vi "Autonomous Independent.vi"() -> ()   [LabVIEW 2023]
doc: "This VI is called when autonomous begins, and will automatically be terminated when autonomous ends. You can carry out timed or sensor driven robot movement independently without needing to return to the caller."
uses:
  <vilib>/Rock Robotics/WPI/ThirdParty/REV Robotics/REVLib/Typedef/Spark MAX Idle Mode.ctl
  <vilib>/Rock Robotics/WPI/SafetyOutput/WPI_SafetyOutputConfigMenu.ctl
  <vilib>/Rock Robotics/Network Tables/NT Read String.vi
  <vilib>/Rock Robotics/WPI/Utilities/WPI_GetSetVariantRefNum.vi
panel:
  out "Numeric 2":i32
  in  "Numeric":i32
  out "Sensor Position 8":dbl
  out "Sensor Position 7":dbl
  out "?":dbl
  out "Sensor Position 6":dbl
  out "Sensor Position 5":dbl
  out "Sensor Position 4":dbl
  out "Sensor Position 3":dbl
  out "Sensor Position 2":dbl
  out "Sensor Position":dbl
  out "?":dbl
  # "Autonomous Independent.viBe sure to right-click and choose Data Operations>>Make Current Value default if you want to save the array values with the VI"
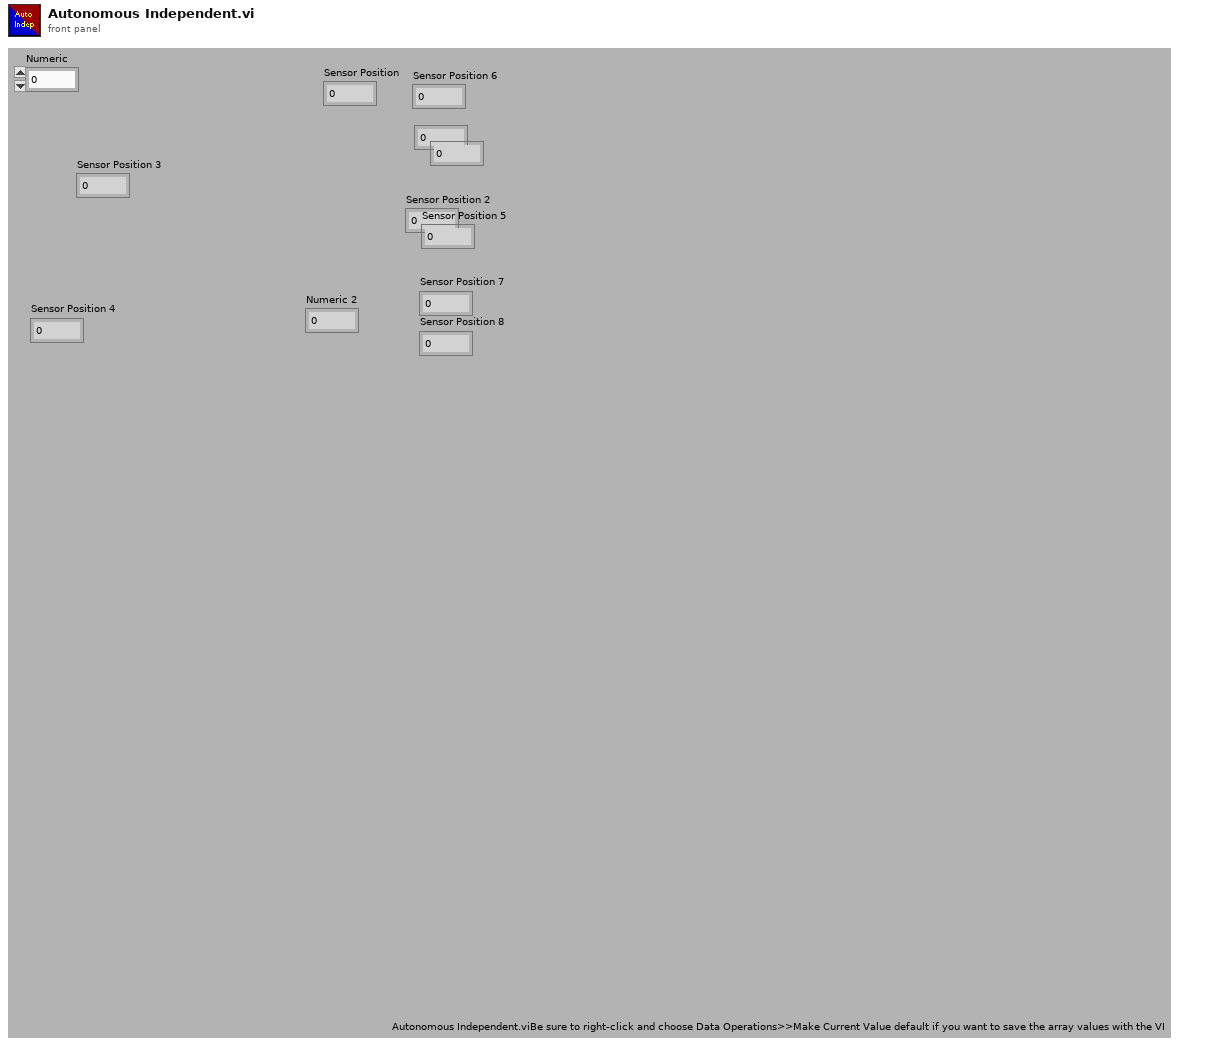
[diagram p1: front panel]
types:
  T1 = typedef "WPI_SafetyOutputConfigMenu.ctl" = enum16{"Enable", "Disable"}
  T2 = enum16{"ação 1", "ação 2", "ação 3", "ação 4", "ação 5", "ação 7", "ação 8"}
  T3 = typedef "Spark MAX Idle Mode.ctl" = enum16{"Coast", "Brake"}
  T4 = enum16{"ação 1", "ação 2", "ação 3", "ação 4", "ação 5"}
  T5 = typedef "WPI_RobotDriveDevRef.ctl" = cluster{"DevStatus":errorcluster, "Motors[]":T6[], "Square Inputs":bool, "Max Output":dbl}
  T6 = typedef "WPI_MotorControlDeviceRef.ctl" = cluster{"DeviceStatus":errorcluster, "Type":T7, "PWM":cluster{"PWM Channel":T8, "DeadBand":T9}, "CAN":cluster{"Device Number":u8, "SetOutput VI Ref":variant, "GetOutput VI Ref":variant, "Enable VI Ref":variant, "Disable VI Ref":variant, "Data":variant}, "Invert":bool, "DIO PWM":cluster{"PWM \"Enable\" Channel":T8, "DIOChannel":T10, "PWM Rate":dbl}}
  T7 = typedef "WPI_MotorControlType.ctl" = enum16{"PWM", "CAN", "DIO PWM"}
  T8 = typedef "FPGA_DIOPWMChannel.ctl" = enum8{"PWM 0", "PWM 1", "PWM 2", "PWM 3", "PWM 4", "PWM 5", "PWM 6", "PWM 7", "PWM 8", "PWM 9", "PWM MXP 0", "PWM MXP 1", "PWM MXP 2", "PWM MXP 3", "PWM MXP 4", "PWM MXP 5", "PWM MXP 6", "PWM MXP 7", "PWM MXP 8", "PWM MXP 9", "Invalid"}
  T9 = typedef "WPI_PWMDeadband.ctl" = cluster{"Name":string, "maxPositivePwm":i32, "minPositivePwm":i32, "centerPwm":i32, "maxNegativePwm":i32, "minNegativePwm":i32, "angularRange":u16}
  T10 = typedef "FPGA_DIOChannel.ctl" = enum8{"DIO 0", "DIO 1", "DIO 2", "DIO 3", "DIO 4", "DIO 5", "DIO 6", "DIO 7", "DIO 8", "DIO 9", "DIO MXP 0", "DIO MXP 1", "DIO MXP 2", "DIO MXP 3", "DIO MXP 4", "DIO MXP 5", "DIO MXP 6", "DIO MXP 7", "DIO MXP 8", "DIO MXP 9", "DIO MXP 10", "DIO MXP 11", "DIO MXP 12", "DIO MXP 13", "DIO MXP 14", "DIO MXP 15", "SPI Port CS1", "SPI Port CS2", "SPI Port CS3", "SPI Port MISO", "SPI Port MOSI", "Invalid"}
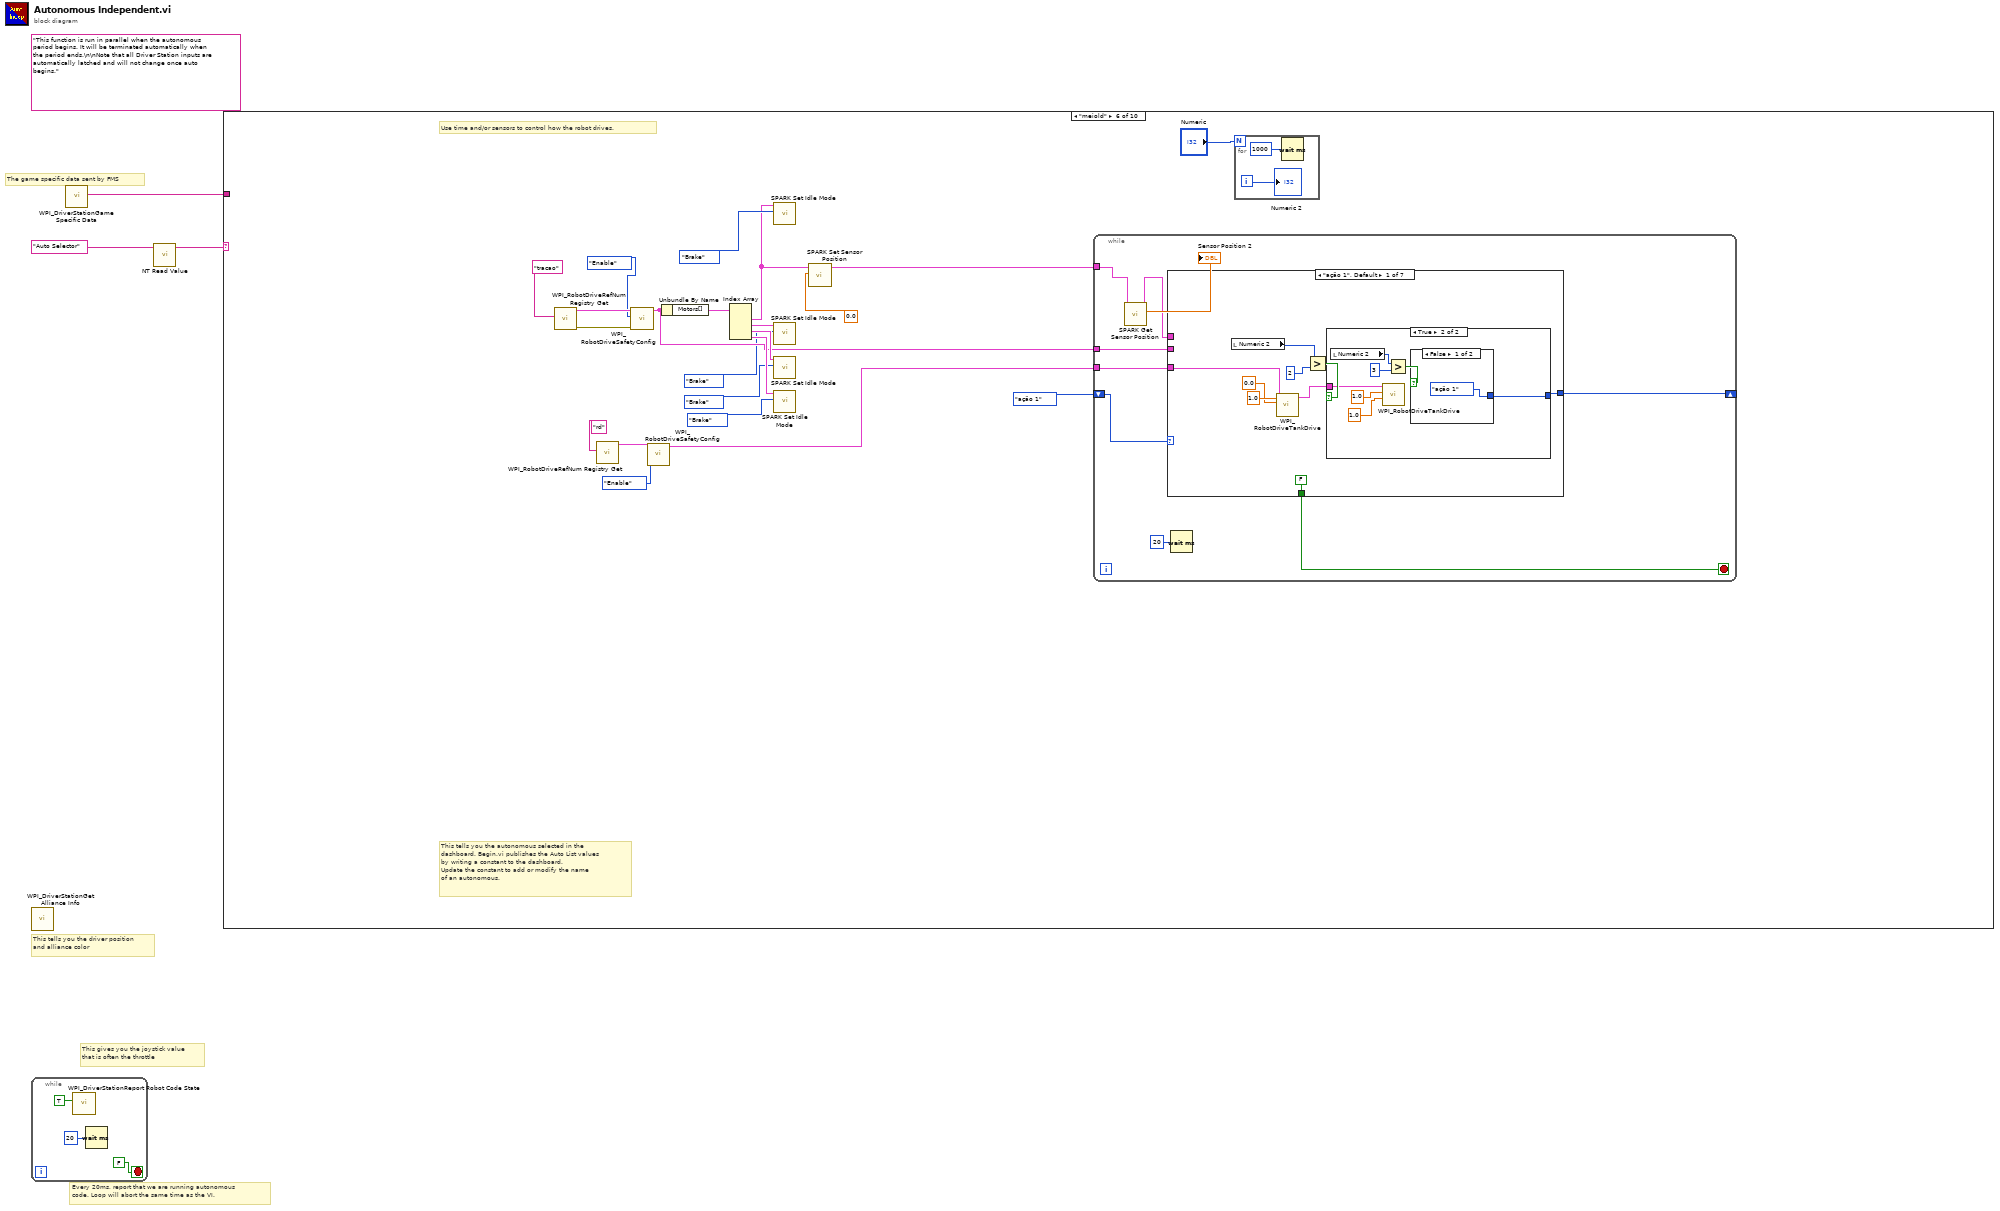
[diagram p0: block diagram]
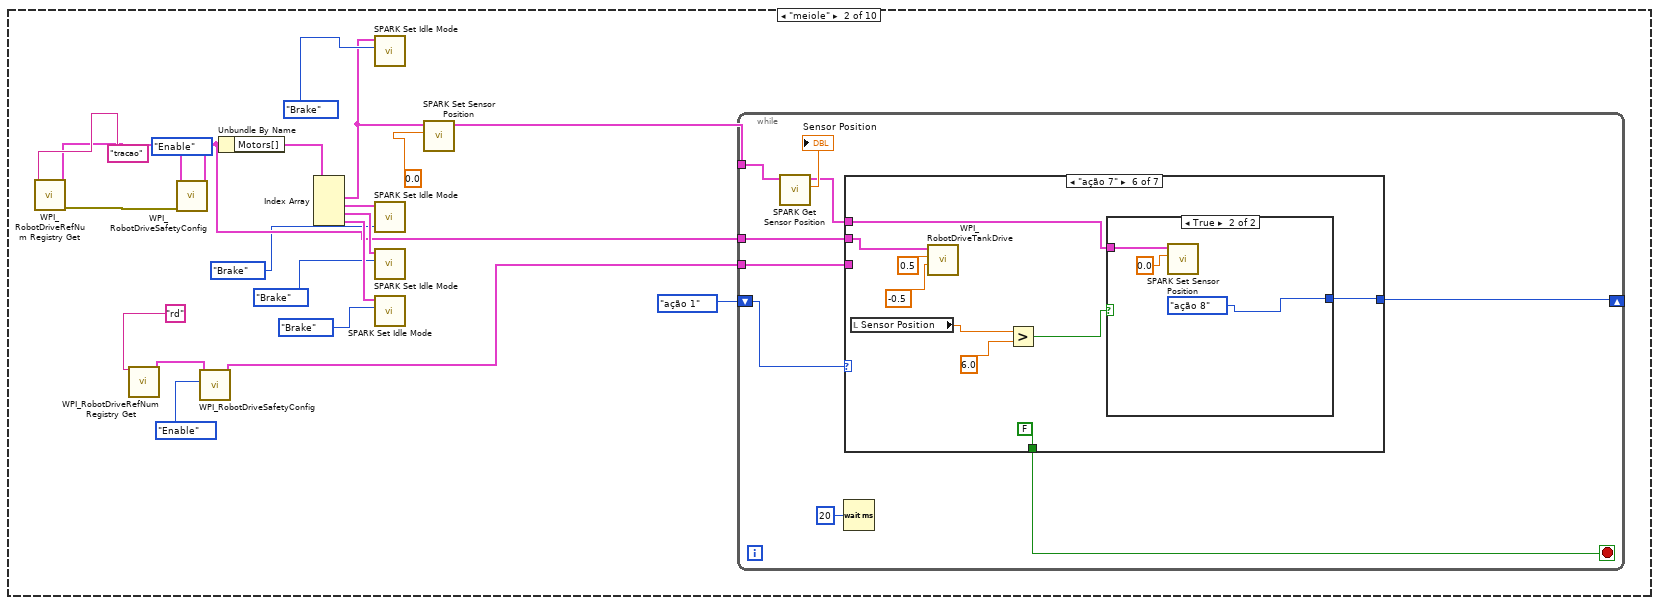
[diagram p3: hidden frame]
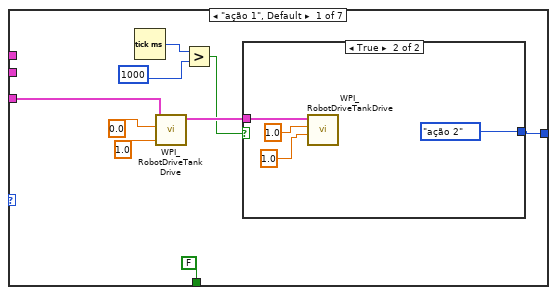
[diagram p4: hidden frame]
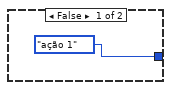
[diagram p5: hidden frame]
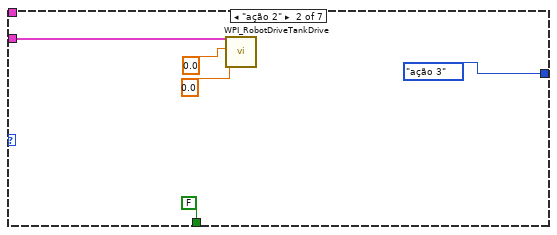
[diagram p6: hidden frame]
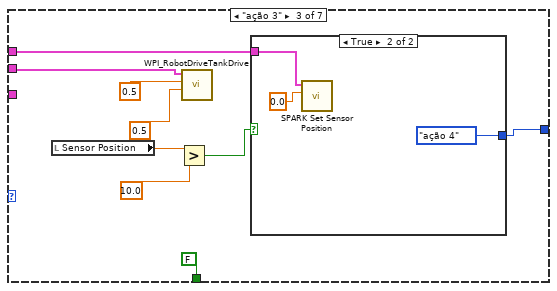
[diagram p7: hidden frame]
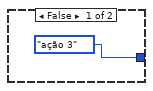
[diagram p8: hidden frame]
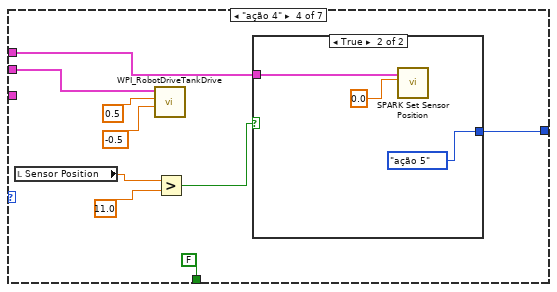
[diagram p9: hidden frame]
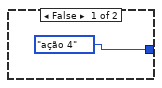
[diagram p10: hidden frame]
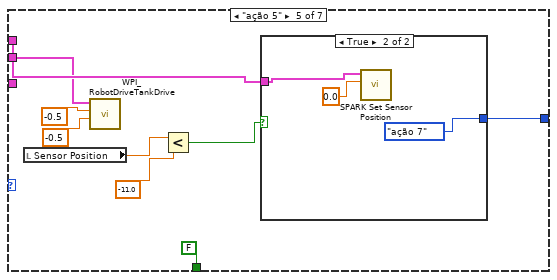
[diagram p11: hidden frame]
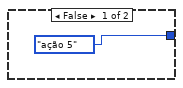
[diagram p12: hidden frame]
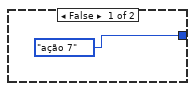
[diagram p13: hidden frame]
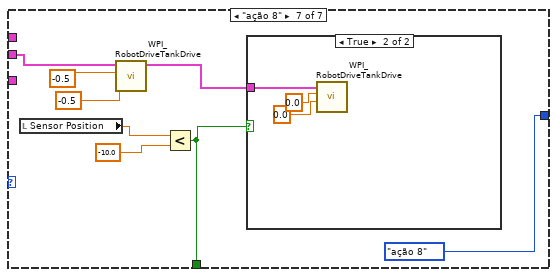
[diagram p14: hidden frame]
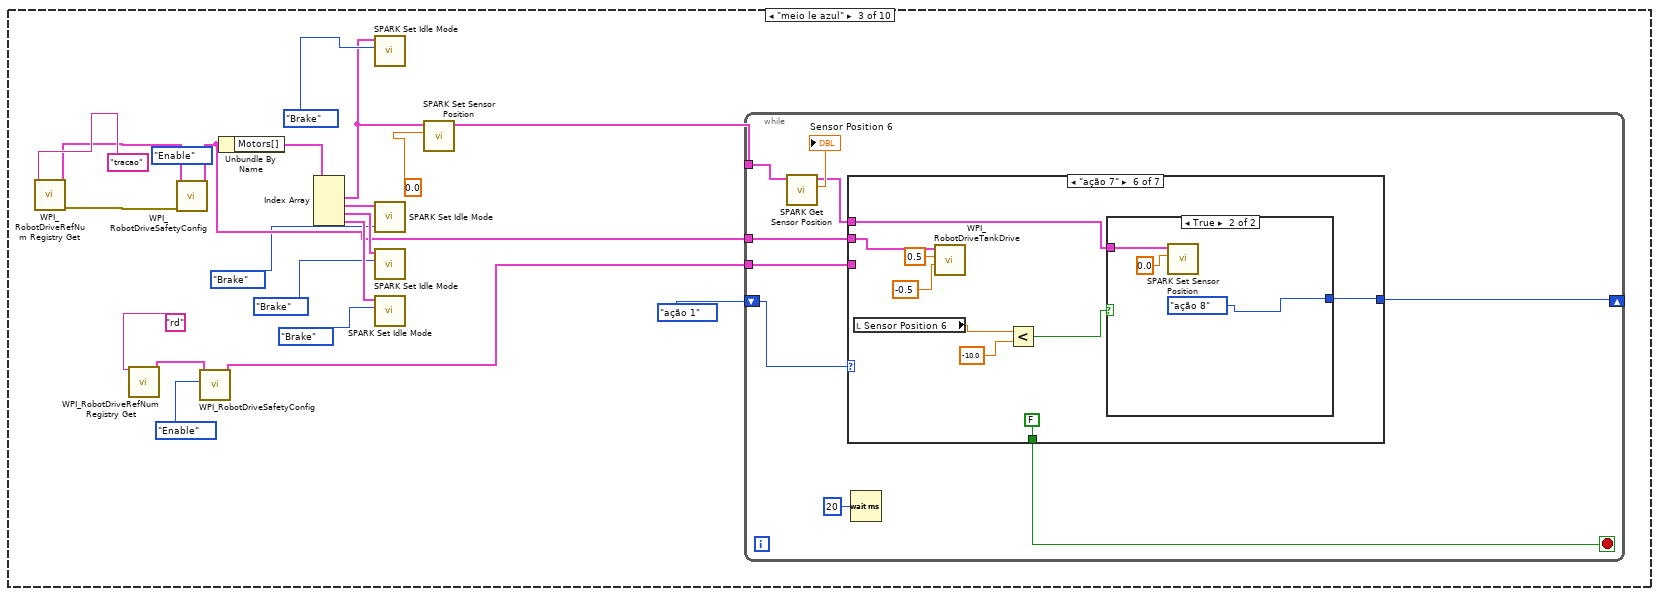
[diagram p16: hidden frame]
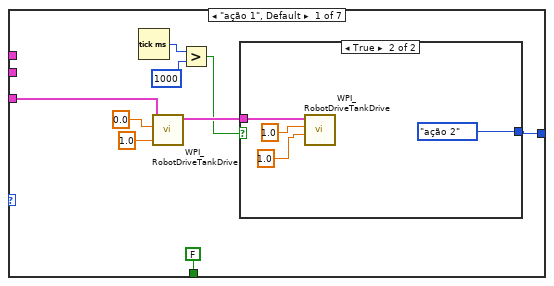
[diagram p17: hidden frame]
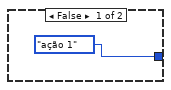
[diagram p18: hidden frame]
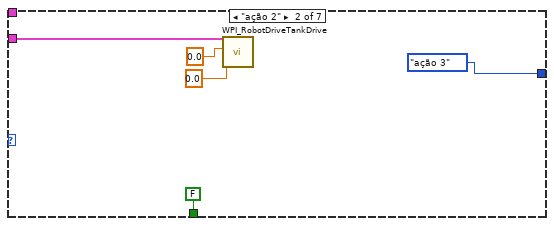
[diagram p19: hidden frame]
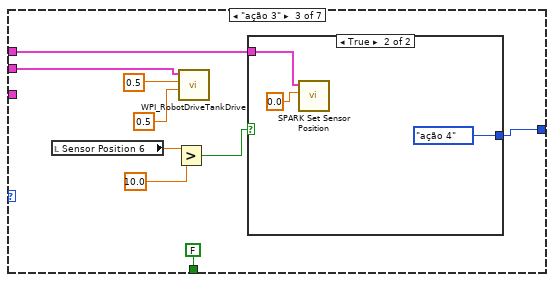
[diagram p20: hidden frame]
diagram:
  (unwired) "This function is run in parallel when the autonomous period begins. It will be terminated automatically when the period ends.\n\nNote that all Driver Station inputs are automatically latched and will not change once auto begins."
  # "The game specific data sent by FMS"
  # "This tells you the autonomous selected in the \ndashboard. Begin.vi publishes the Auto List values\nby writing a constant to the dashboard.\nUpdate the constant to add or modify the name\nof an autonomous."
  # "Every 20ms, report that we are running autonomous\ncode. Loop will abort the same time as the VI."
  # "This gives you the joystick value\nthat is often the throttle"
  # "Use time and/or sensors to control how the robot drives."
  # "This tells you the driver position\nand alliance color"
  n1 = call <vilib>:"WPI_DriverStationGet Alliance Info.vi"() -> ()  [unwired: 12 out]
  n2 = while {
    stop <- FALSE stop-if-true
    n3 = call <vilib>:"WPI_DriverStationReport Robot Code State.vi"("Autonomous"=TRUE) -> ()  [unwired: 10 in, 1 out]
    n4 = Wait (ms)(milliseconds to wait=u32 20) -> ()  [unwired: 1 out]
  }
  n5 = call <vilib>:"WPI_DriverStationGame Specific Data.vi"() -> ("Game Specific Data"=w1:string)  [unwired: 11 in]
  n6 = call-poly <vilib>:"NT Read Value.vi"("name"="Auto Selector" ("Name")) -> ("value"=w2:string)  [unwired: 8 in, 2 out]
  n7 = case shown="\"meiold\"" w2 {
    tunnel: w1 -> [_ _ _ _ _ _ _ _ _ _]
    frame Default {
    }
    frame "meiole" {
      n8 = call <vilib>:"WPI_RobotDriveRefNum Registry Get.vi"("refnum name"="tracao") -> ("error out"=w26:errorcluster, "RobotDriveDevRef"=w25:T5)  [unwired: 9 in]
      n9 = call <vilib>:"WPI_RobotDriveRefNum Registry Get.vi"("refnum name"="rd") -> ("RobotDriveDevRef"=w15:T5)  [unwired: 9 in, 1 out]
      n10 = call <vilib>:"WPI_RobotDriveSafetyConfig.vi"("error in (no error)"=w26, "mode"=WPI_SafetyOutputConfigMenu."Enable", "RobotDriveDevRef"=w25) -> ("RobotDriveDevRef"=w13:T5)  [unwired: 7 in, 1 out]
      n11 = call <vilib>:"WPI_RobotDriveSafetyConfig.vi"("mode"=WPI_SafetyOutputConfigMenu."Enable", "RobotDriveDevRef"=w15) -> ("RobotDriveDevRef"=w14:T5)  [unwired: 8 in, 1 out]
      n12 = Unbundle By Name(w13) -> ("Motors[]"=w24:T6[])
      n13 = Index Array(array=w24) -> (element #1=w17:T6, element #2=w21:T6, element #3=w20:T6, element #4=w19:T6)  [unwired: 4 in]
      n14 = call <vilib>:"SPARK Set Idle Mode.vi"("Idle Mode"=Spark_MAX_Idle_Mode."Brake", "MotorControlDeviceRef in"=w17) -> ()  [unwired: 8 in, 2 out]
      n15 = call <vilib>:"SPARK Set Idle Mode.vi"("Idle Mode"=Spark_MAX_Idle_Mode."Brake", "MotorControlDeviceRef in"=w21) -> ()  [unwired: 8 in, 2 out]
      n16 = call <vilib>:"SPARK Set Idle Mode.vi"("Idle Mode"=Spark_MAX_Idle_Mode."Brake", "MotorControlDeviceRef in"=w20) -> ()  [unwired: 8 in, 2 out]
      n17 = call <vilib>:"SPARK Set Idle Mode.vi"("Idle Mode"=Spark_MAX_Idle_Mode."Brake", "MotorControlDeviceRef in"=w19) -> ()  [unwired: 8 in, 2 out]
      n18 = call <vilib>:"SPARK Set Sensor Position.vi"("Position"=0.0, "MotorControlDeviceRef"=w17) -> ("MotorControlDeviceRef"=w12:T6)  [unwired: 8 in, 1 out]
      n19 = while {
        shift-right: [w33] -> _
        shift-left: T2."ação 1" -> [w35]
        tunnel: w14 -> [w34]
        tunnel: w13 -> [w32]
        tunnel: w12 -> [w30]
        stop <- w28 stop-if-true
        n20 = call <vilib>:"SPARK Get Sensor Position.vi"("MotorControlDevRef in"=w30) -> ("Sensor Position"=→"Sensor Position":dbl, "MotorControlDevRef out"=w29:T6)  [unwired: 7 in, 2 out]
        n21 = Wait (ms)(milliseconds to wait=u32 20) -> ()  [unwired: 1 out]
        n22 = case shown="\"ação 7\"" w35 {
          tunnel: w34 -> [w43 w55 _ _ _ _ _]
          tunnel: [w38 T2."ação 3" w57 w70 w83 w96 T2."ação 8"] -> w33
          tunnel: w32 -> [_ _ w64 w77 w87 w103 w115]
          tunnel: w29 -> [_ _ w58 w71 w90 w97 _]
          tunnel: [FALSE FALSE FALSE FALSE FALSE FALSE w109] -> w28
          frame "ação 1", Default {
            n23 = Tick Count (ms)() -> (millisecond timer value=w41:u32)
            n24 = call <vilib>:"WPI_RobotDriveTankDrive.vi"("Right axis value"=1.0, "Left axis value"=0.0, "RobotDriveDevRef"=w43) -> ("RobotDriveDevRef"=w42:T5)  [unwired: 6 in, 2 out]
            n25 = Greater?(x=w41, y=u32 1000) -> (0:w39:bool)
            n26 = case shown="True" w39 {
              tunnel: w42 -> [_ w48]
              tunnel: [T2."ação 1" T2."ação 2"] -> w38
              frame False {
              }
              frame True {
                n27 = call <vilib>:"WPI_RobotDriveTankDrive.vi"("Right axis value"=1.0 ("Left axis value"), "Left axis value"=1.0 ("Right axis value"), "RobotDriveDevRef"=w48) -> ()  [unwired: 6 in, 3 out]
              }
            }
          }
          frame "ação 2" {
            n28 = call <vilib>:"WPI_RobotDriveTankDrive.vi"("Right axis value"=0.0, "Left axis value"=0.0, "RobotDriveDevRef"=w55) -> ()  [unwired: 6 in, 3 out]
          }
          frame "ação 3" {
            n29 = local read "Sensor Position"() -> (w60:dbl)
            n30 = Greater?(x=w60, y=10.0) -> (0:w61:bool)
            n31 = call <vilib>:"WPI_RobotDriveTankDrive.vi"("Right axis value"=0.5 ("Left axis value"), "Left axis value"=0.5, "RobotDriveDevRef"=w64) -> ()  [unwired: 6 in, 3 out]
            n32 = case shown="True" w61 {
              tunnel: w58 -> [_ w68]
              tunnel: [T2."ação 3" T2."ação 4"] -> w57
              frame False {
              }
              frame True {
                n33 = call <vilib>:"SPARK Set Sensor Position.vi"("Position"=0.0, "MotorControlDeviceRef"=w68) -> ()  [unwired: 8 in, 2 out]
              }
            }
          }
          frame "ação 4" {
            n34 = local read "Sensor Position"() -> (w74:dbl)
            n35 = call <vilib>:"WPI_RobotDriveTankDrive.vi"("Right axis value"=-0.5 ("Left axis value"), "Left axis value"=0.5, "RobotDriveDevRef"=w77) -> ()  [unwired: 6 in, 3 out]
            n36 = Greater?(x=w74, y=11.0) -> (0:w72:bool)
            n37 = case shown="True" w72 {
              tunnel: w71 -> [_ w81]
              tunnel: [T2."ação 4" T2."ação 5"] -> w70
              frame False {
              }
              frame True {
                n38 = call <vilib>:"SPARK Set Sensor Position.vi"("Position"=0.0, "MotorControlDeviceRef"=w81) -> ()  [unwired: 8 in, 2 out]
              }
            }
          }
          frame "ação 5" {
            n39 = local read "Sensor Position"() -> (w86:dbl)
            n40 = call <vilib>:"WPI_RobotDriveTankDrive.vi"("Right axis value"=-0.5 ("Left axis value"), "Left axis value"=-0.5, "RobotDriveDevRef"=w87) -> ()  [unwired: 6 in, 3 out]
            n41 = Less?(x=w86, y=-11.0) -> (x < y?=w84:bool)
            n42 = case shown="True" w84 {
              tunnel: w90 -> [_ w93]
              tunnel: [T2."ação 5" T2."ação 7"] -> w83
              frame False {
              }
              frame True {
                n43 = call <vilib>:"SPARK Set Sensor Position.vi"("Position"=0.0, "MotorControlDeviceRef"=w93) -> ()  [unwired: 8 in, 2 out]
              }
            }
          }
          frame "ação 7" {
            n44 = local read "Sensor Position"() -> (w100:dbl)
            n45 = call <vilib>:"WPI_RobotDriveTankDrive.vi"("Right axis value"=-0.5 ("Left axis value"), "Left axis value"=0.5, "RobotDriveDevRef"=w103) -> ()  [unwired: 6 in, 3 out]
            n46 = Greater?(x=w100, y=6.0) -> (0:w98:bool)
            n47 = case shown="True" w98 {
              tunnel: w97 -> [_ w107]
              tunnel: [T2."ação 7" T2."ação 8"] -> w96
              frame False {
              }
              frame True {
                n48 = call <vilib>:"SPARK Set Sensor Position.vi"("Position"=0.0, "MotorControlDeviceRef"=w107) -> ()  [unwired: 8 in, 2 out]
              }
            }
          }
          frame "ação 8" {
            n49 = local read "Sensor Position"() -> (w112:dbl)
            n50 = call <vilib>:"WPI_RobotDriveTankDrive.vi"("Right axis value"=-0.5 ("Left axis value"), "Left axis value"=-0.5, "RobotDriveDevRef"=w115) -> ("RobotDriveDevRef"=w110:T5)  [unwired: 6 in, 2 out]
            n51 = Less?(x=w112, y=-10.0) -> (x < y?=w109:bool)
            n52 = case shown="True" w109 {
              tunnel: w110 -> [_ w118]
              frame False {
              }
              frame True {
                n53 = call <vilib>:"WPI_RobotDriveTankDrive.vi"("Right axis value"=0.0 ("Left axis value"), "Left axis value"=0.0, "RobotDriveDevRef"=w118) -> ()  [unwired: 6 in, 3 out]
              }
            }
          }
        }
      }
    }
    frame "meio le azul" {
      n54 = call <vilib>:"WPI_RobotDriveRefNum Registry Get.vi"("refnum name"="tracao") -> ("error out"=w138:errorcluster, "RobotDriveDevRef"=w137:T5)  [unwired: 9 in]
      n55 = call <vilib>:"WPI_RobotDriveRefNum Registry Get.vi"("refnum name"="rd") -> ("RobotDriveDevRef"=w127:T5)  [unwired: 9 in, 1 out]
      n56 = call <vilib>:"WPI_RobotDriveSafetyConfig.vi"("error in (no error)"=w138, "mode"=WPI_SafetyOutputConfigMenu."Enable", "RobotDriveDevRef"=w137) -> ("RobotDriveDevRef"=w125:T5)  [unwired: 7 in, 1 out]
      n57 = call <vilib>:"WPI_RobotDriveSafetyConfig.vi"("mode"=WPI_SafetyOutputConfigMenu."Enable", "RobotDriveDevRef"=w127) -> ("RobotDriveDevRef"=w126:T5)  [unwired: 8 in, 1 out]
      n58 = Unbundle By Name(w125) -> ("Motors[]"=w136:T6[])
      n59 = Index Array(array=w136) -> (element #1=w129:T6, element #2=w133:T6, element #3=w132:T6, element #4=w131:T6)  [unwired: 4 in]
      n60 = call <vilib>:"SPARK Set Idle Mode.vi"("Idle Mode"=Spark_MAX_Idle_Mode."Brake", "MotorControlDeviceRef in"=w129) -> ()  [unwired: 8 in, 2 out]
      n61 = call <vilib>:"SPARK Set Idle Mode.vi"("Idle Mode"=Spark_MAX_Idle_Mode."Brake", "MotorControlDeviceRef in"=w133) -> ()  [unwired: 8 in, 2 out]
      n62 = call <vilib>:"SPARK Set Idle Mode.vi"("Idle Mode"=Spark_MAX_Idle_Mode."Brake", "MotorControlDeviceRef in"=w132) -> ()  [unwired: 8 in, 2 out]
      n63 = call <vilib>:"SPARK Set Idle Mode.vi"("Idle Mode"=Spark_MAX_Idle_Mode."Brake", "MotorControlDeviceRef in"=w131) -> ()  [unwired: 8 in, 2 out]
      n64 = call <vilib>:"SPARK Set Sensor Position.vi"("Position"=0.0, "MotorControlDeviceRef"=w129) -> ("MotorControlDeviceRef"=w124:T6)  [unwired: 8 in, 1 out]
      n65 = while {
        shift-right: [w145] -> _
        shift-left: T2."ação 1" -> [w147]
        tunnel: w126 -> [w146]
        tunnel: w125 -> [w144]
        tunnel: w124 -> [w142]
        stop <- w140 stop-if-true
        n66 = call <vilib>:"SPARK Get Sensor Position.vi"("MotorControlDevRef in"=w142) -> ("Sensor Position"=→"Sensor Position 6":dbl, "MotorControlDevRef out"=w141:T6)  [unwired: 7 in, 2 out]
        n67 = case shown="\"ação 7\"" w147 {
          tunnel: w146 -> [w155 w167 _ _ _ _ _]
          tunnel: [w150 T2."ação 3" w169 w182 w195 w208 T2."ação 8"] -> w145
          tunnel: w144 -> [_ _ w176 w189 w199 w215 w227]
          tunnel: w141 -> [_ _ w170 w183 w202 w209 _]
          tunnel: [FALSE FALSE FALSE FALSE FALSE FALSE w221] -> w140
          frame "ação 1", Default {
            n68 = Tick Count (ms)() -> (millisecond timer value=w153:u32)
            n69 = call <vilib>:"WPI_RobotDriveTankDrive.vi"("Right axis value"=1.0, "Left axis value"=0.0, "RobotDriveDevRef"=w155) -> ("RobotDriveDevRef"=w154:T5)  [unwired: 6 in, 2 out]
            n70 = Greater?(x=w153, y=u32 1000) -> (0:w151:bool)
            n71 = case shown="True" w151 {
              tunnel: w154 -> [_ w160]
              tunnel: [T2."ação 1" T2."ação 2"] -> w150
              frame False {
              }
              frame True {
                n72 = call <vilib>:"WPI_RobotDriveTankDrive.vi"("Right axis value"=1.0 ("Left axis value"), "Left axis value"=1.0 ("Right axis value"), "RobotDriveDevRef"=w160) -> ()  [unwired: 6 in, 3 out]
              }
            }
          }
          frame "ação 2" {
            n73 = call <vilib>:"WPI_RobotDriveTankDrive.vi"("Right axis value"=0.0, "Left axis value"=0.0, "RobotDriveDevRef"=w167) -> ()  [unwired: 6 in, 3 out]
          }
          frame "ação 3" {
            n74 = local read "Sensor Position 6"() -> (w172:dbl)
            n75 = Greater?(x=w172, y=10.0) -> (0:w173:bool)
            n76 = call <vilib>:"WPI_RobotDriveTankDrive.vi"("Right axis value"=0.5 ("Left axis value"), "Left axis value"=0.5, "RobotDriveDevRef"=w176) -> ()  [unwired: 6 in, 3 out]
            n77 = case shown="True" w173 {
              tunnel: w170 -> [_ w180]
              tunnel: [T2."ação 3" T2."ação 4"] -> w169
              frame False {
              }
              frame True {
                n78 = call <vilib>:"SPARK Set Sensor Position.vi"("Position"=0.0, "MotorControlDeviceRef"=w180) -> ()  [unwired: 8 in, 2 out]
              }
            }
          }
          frame "ação 4" {
            n79 = local read "Sensor Position 6"() -> (w186:dbl)
            n80 = call <vilib>:"WPI_RobotDriveTankDrive.vi"("Right axis value"=-0.5 ("Left axis value"), "Left axis value"=0.5, "RobotDriveDevRef"=w189) -> ()  [unwired: 6 in, 3 out]
            n81 = Less?(x=w186, y=-10.0) -> (x < y?=w184:bool)
            n82 = case shown="True" w184 {
              tunnel: w183 -> [_ w193]
              tunnel: [T2."ação 4" T2."ação 5"] -> w182
              frame False {
              }
              frame True {
                n83 = call <vilib>:"SPARK Set Sensor Position.vi"("Position"=0.0, "MotorControlDeviceRef"=w193) -> ()  [unwired: 8 in, 2 out]
              }
            }
          }
          frame "ação 5" {
            n84 = local read "Sensor Position 6"() -> (w198:dbl)
            n85 = call <vilib>:"WPI_RobotDriveTankDrive.vi"("Right axis value"=-0.5 ("Left axis value"), "Left axis value"=-0.5, "RobotDriveDevRef"=w199) -> ()  [unwired: 6 in, 3 out]
            n86 = Less?(x=w198, y=-13.0) -> (x < y?=w196:bool)
            n87 = case shown="True" w196 {
              tunnel: w202 -> [_ w205]
              tunnel: [T2."ação 5" T2."ação 7"] -> w195
              frame False {
              }
              frame True {
                n88 = call <vilib>:"SPARK Set Sensor Position.vi"("Position"=0.0, "MotorControlDeviceRef"=w205) -> ()  [unwired: 8 in, 2 out]
              }
            }
          }
          frame "ação 7" {
            n89 = local read "Sensor Position 6"() -> (w212:dbl)
            n90 = call <vilib>:"WPI_RobotDriveTankDrive.vi"("Right axis value"=-0.5 ("Left axis value"), "Left axis value"=0.5, "RobotDriveDevRef"=w215) -> ()  [unwired: 6 in, 3 out]
            n91 = Less?(x=w212, y=-10.0) -> (x < y?=w210:bool)
            n92 = case shown="True" w210 {
              tunnel: w209 -> [_ w219]
              tunnel: [T2."ação 7" T2."ação 8"] -> w208
              frame False {
              }
              frame True {
                n93 = call <vilib>:"SPARK Set Sensor Position.vi"("Position"=0.0, "MotorControlDeviceRef"=w219) -> ()  [unwired: 8 in, 2 out]
              }
            }
          }
          frame "ação 8" {
            n94 = local read "Sensor Position 6"() -> (w224:dbl)
            n95 = call <vilib>:"WPI_RobotDriveTankDrive.vi"("Right axis value"=-0.5 ("Left axis value"), "Left axis value"=-0.5, "RobotDriveDevRef"=w227) -> ("RobotDriveDevRef"=w222:T5)  [unwired: 6 in, 2 out]
            n96 = Less?(x=w224, y=-30.0) -> (x < y?=w221:bool)
            n97 = case shown="True" w221 {
              tunnel: w222 -> [_ w230]
              frame False {
              }
              frame True {
                n98 = call <vilib>:"WPI_RobotDriveTankDrive.vi"("Right axis value"=0.0 ("Left axis value"), "Left axis value"=0.0, "RobotDriveDevRef"=w230) -> ()  [unwired: 6 in, 3 out]
              }
            }
          }
        }
        n99 = Wait (ms)(milliseconds to wait=u32 20) -> ()  [unwired: 1 out]
      }
    }
    frame "direita" {
      n100 = call <vilib>:"WPI_RobotDriveRefNum Registry Get.vi"("refnum name"="rd") -> ("RobotDriveDevRef"=w233:T5)  [unwired: 9 in, 1 out]
      n101 = call <vilib>:"WPI_RobotDriveRefNum Registry Get.vi"("refnum name"="tracao") -> ("error out"=w250:errorcluster, "RobotDriveDevRef"=w249:T5)  [unwired: 9 in]
      n102 = call <vilib>:"WPI_RobotDriveSafetyConfig.vi"("mode"=WPI_SafetyOutputConfigMenu."Enable", "RobotDriveDevRef"=w233) -> ("RobotDriveDevRef"=w232:T5)  [unwired: 8 in, 1 out]
      n103 = call <vilib>:"WPI_RobotDriveSafetyConfig.vi"("error in (no error)"=w250, "mode"=WPI_SafetyOutputConfigMenu."Enable", "RobotDriveDevRef"=w249) -> ("RobotDriveDevRef"=w235:T5)  [unwired: 7 in, 1 out]
      n104 = Unbundle By Name(w235) -> ("Motors[]"=w247:T6[])
      n105 = Index Array(array=w247) -> (element #1=w239:T6, element #2=w242:T6, element #3=w241:T6, element #4=w240:T6)  [unwired: 4 in]
      n106 = call <vilib>:"SPARK Set Idle Mode.vi"("Idle Mode"=Spark_MAX_Idle_Mode."Brake", "MotorControlDeviceRef in"=w239) -> ()  [unwired: 8 in, 2 out]
      n107 = call <vilib>:"SPARK Set Idle Mode.vi"("Idle Mode"=Spark_MAX_Idle_Mode."Brake", "MotorControlDeviceRef in"=w242) -> ()  [unwired: 8 in, 2 out]
      n108 = call <vilib>:"SPARK Set Idle Mode.vi"("Idle Mode"=Spark_MAX_Idle_Mode."Brake", "MotorControlDeviceRef in"=w241) -> ()  [unwired: 8 in, 2 out]
      n109 = call <vilib>:"SPARK Set Idle Mode.vi"("Idle Mode"=Spark_MAX_Idle_Mode."Brake", "MotorControlDeviceRef in"=w240) -> ()  [unwired: 8 in, 2 out]
      n110 = call <vilib>:"SPARK Set Sensor Position.vi"("Position"=0.0, "MotorControlDeviceRef"=w239) -> ("MotorControlDeviceRef"=w237:T6)  [unwired: 8 in, 1 out]
      n111 = while {
        shift-right: [w254] -> _
        shift-left: T4."ação 1" -> [w259]
        tunnel: w237 -> [w257]
        tunnel: w235 -> [w255]
        tunnel: w232 -> [w253]
        stop <- w258 stop-if-true
        n112 = call <vilib>:"SPARK Get Sensor Position.vi"("MotorControlDevRef in"=w257) -> ("Sensor Position"=→"?":dbl, "MotorControlDevRef out"=w252:T6)  [unwired: 7 in, 2 out]
        n113 = case shown="\"ação 3\"" w259 {
          tunnel: [FALSE FALSE FALSE FALSE w309] -> w258
          tunnel: [w262 T4."ação 3" w281 w294 T4."ação 5"] -> w254
          tunnel: w255 -> [_ _ w283 w296 w306]
          tunnel: w253 -> [w261 w275 _ _ _]
          tunnel: w252 -> [_ _ w280 w293 _]
          frame "ação 1", Default {
            n114 = Tick Count (ms)() -> (millisecond timer value=w266:u32)
            n115 = call <vilib>:"WPI_RobotDriveTankDrive.vi"("Right axis value"=1.0, "Left axis value"=0.0, "RobotDriveDevRef"=w261) -> ("RobotDriveDevRef"=w267:T5)  [unwired: 6 in, 2 out]
            n116 = Greater?(x=w266, y=u32 1000) -> (0:w264:bool)
            n117 = case shown="True" w264 {
              tunnel: w267 -> [_ w272]
              tunnel: [T4."ação 1" T4."ação 2"] -> w262
              frame False {
              }
              frame True {
                n118 = call <vilib>:"WPI_RobotDriveTankDrive.vi"("Right axis value"=1.0 ("Left axis value"), "Left axis value"=1.0 ("Right axis value"), "RobotDriveDevRef"=w272) -> ()  [unwired: 6 in, 3 out]
              }
            }
          }
          frame "ação 2" {
            n119 = call <vilib>:"WPI_RobotDriveTankDrive.vi"("Right axis value"=0.0 ("Left axis value"), "Left axis value"=0.0, "RobotDriveDevRef"=w275) -> ()  [unwired: 6 in, 3 out]
          }
          frame "ação 3" {
            n120 = local read item#?() -> (w282:dbl)
            n121 = Greater?(x=w282, y=12.5) -> (0:w286:bool)
            n122 = call <vilib>:"WPI_RobotDriveTankDrive.vi"("Right axis value"=0.5 ("Left axis value"), "Left axis value"=0.5, "RobotDriveDevRef"=w283) -> ()  [unwired: 6 in, 3 out]
            n123 = case shown="True" w286 {
              tunnel: [T4."ação 3" T4."ação 4"] -> w281
              tunnel: w280 -> [_ w290]
              frame False {
              }
              frame True {
                n124 = call <vilib>:"SPARK Set Sensor Position.vi"("Position"=0.0, "MotorControlDeviceRef"=w290) -> ()  [unwired: 8 in, 2 out]
              }
            }
          }
          frame "ação 4" {
            n125 = local read item#?() -> (w295:dbl)
            n126 = call <vilib>:"WPI_RobotDriveTankDrive.vi"("Right axis value"=-0.5 ("Left axis value"), "Left axis value"=0.5, "RobotDriveDevRef"=w296) -> ()  [unwired: 6 in, 3 out]
            n127 = Greater?(x=w295, y=12.0) -> (0:w298:bool)
            n128 = case shown="True" w298 {
              tunnel: [T4."ação 4" T4."ação 5"] -> w294
              tunnel: w293 -> [_ w303]
              frame False {
              }
              frame True {
                n129 = call <vilib>:"SPARK Set Sensor Position.vi"("Position"=0.0, "MotorControlDeviceRef"=w303) -> ()  [unwired: 8 in, 2 out]
              }
            }
          }
          frame "ação 5" {
            n130 = local read item#?() -> (w308:dbl)
            n131 = call <vilib>:"WPI_RobotDriveTankDrive.vi"("Right axis value"=-0.5 ("Left axis value"), "Left axis value"=-0.5, "RobotDriveDevRef"=w306) -> ("RobotDriveDevRef"=w310:T5)  [unwired: 6 in, 2 out]
            n132 = Less?(x=w308, y=-35.0) -> (x < y?=w309:bool)
            n133 = case shown="True" w309 {
              tunnel: w310 -> [_ w314]
              frame False {
              }
              frame True {
                n134 = call <vilib>:"WPI_RobotDriveTankDrive.vi"("Right axis value"=0.0 ("Left axis value"), "Left axis value"=0.0, "RobotDriveDevRef"=w314) -> ()  [unwired: 6 in, 3 out]
              }
            }
          }
        }
        n135 = Wait (ms)(milliseconds to wait=u32 20) -> ()  [unwired: 1 out]
      }
    }
    frame "direita azul" {
      n136 = call <vilib>:"WPI_RobotDriveRefNum Registry Get.vi"("refnum name"="rd") -> ("RobotDriveDevRef"=w319:T5)  [unwired: 9 in, 1 out]
      n137 = call <vilib>:"WPI_RobotDriveRefNum Registry Get.vi"("refnum name"="tracao") -> ("error out"=w336:errorcluster, "RobotDriveDevRef"=w335:T5)  [unwired: 9 in]
      n138 = call <vilib>:"WPI_RobotDriveSafetyConfig.vi"("mode"=WPI_SafetyOutputConfigMenu."Enable", "RobotDriveDevRef"=w319) -> ("RobotDriveDevRef"=w318:T5)  [unwired: 8 in, 1 out]
      n139 = call <vilib>:"WPI_RobotDriveSafetyConfig.vi"("error in (no error)"=w336, "mode"=WPI_SafetyOutputConfigMenu."Enable", "RobotDriveDevRef"=w335) -> ("RobotDriveDevRef"=w321:T5)  [unwired: 7 in, 1 out]
      n140 = Unbundle By Name(w321) -> ("Motors[]"=w333:T6[])
      n141 = Index Array(array=w333) -> (element #1=w325:T6, element #2=w328:T6, element #3=w327:T6, element #4=w326:T6)  [unwired: 4 in]
      n142 = call <vilib>:"SPARK Set Idle Mode.vi"("Idle Mode"=Spark_MAX_Idle_Mode."Brake", "MotorControlDeviceRef in"=w325) -> ()  [unwired: 8 in, 2 out]
      n143 = call <vilib>:"SPARK Set Idle Mode.vi"("Idle Mode"=Spark_MAX_Idle_Mode."Brake", "MotorControlDeviceRef in"=w328) -> ()  [unwired: 8 in, 2 out]
      n144 = call <vilib>:"SPARK Set Idle Mode.vi"("Idle Mode"=Spark_MAX_Idle_Mode."Brake", "MotorControlDeviceRef in"=w327) -> ()  [unwired: 8 in, 2 out]
      n145 = call <vilib>:"SPARK Set Idle Mode.vi"("Idle Mode"=Spark_MAX_Idle_Mode."Brake", "MotorControlDeviceRef in"=w326) -> ()  [unwired: 8 in, 2 out]
      n146 = call <vilib>:"SPARK Set Sensor Position.vi"("Position"=0.0, "MotorControlDeviceRef"=w325) -> ("MotorControlDeviceRef"=w323:T6)  [unwired: 8 in, 1 out]
      n147 = while {
        shift-right: [w340] -> _
        shift-left: T4."ação 1" -> [w345]
        tunnel: w323 -> [w343]
        tunnel: w321 -> [w341]
        tunnel: w318 -> [w339]
        stop <- w344 stop-if-true
        n148 = call <vilib>:"SPARK Get Sensor Position.vi"("MotorControlDevRef in"=w343) -> ("Sensor Position"=→"?":dbl, "MotorControlDevRef out"=w338:T6)  [unwired: 7 in, 2 out]
        n149 = case shown="\"ação 5\"" w345 {
          tunnel: [FALSE FALSE FALSE FALSE w395] -> w344
          tunnel: [w348 T4."ação 3" w367 w380 T4."ação 5"] -> w340
          tunnel: w341 -> [_ _ w369 w382 w392]
          tunnel: w339 -> [w347 w361 _ _ _]
          tunnel: w338 -> [_ _ w366 w379 _]
          frame "ação 1", Default {
            n150 = Tick Count (ms)() -> (millisecond timer value=w352:u32)
            n151 = call <vilib>:"WPI_RobotDriveTankDrive.vi"("Right axis value"=1.0, "Left axis value"=0.0, "RobotDriveDevRef"=w347) -> ("RobotDriveDevRef"=w353:T5)  [unwired: 6 in, 2 out]
            n152 = Greater?(x=w352, y=u32 1000) -> (0:w350:bool)
            n153 = case shown="False" w350 {
              tunnel: w353 -> [_ w358]
              tunnel: [T4."ação 1" T4."ação 2"] -> w348
              frame False {
              }
              frame True {
                n154 = call <vilib>:"WPI_RobotDriveTankDrive.vi"("Right axis value"=1.0 ("Left axis value"), "Left axis value"=1.0 ("Right axis value"), "RobotDriveDevRef"=w358) -> ()  [unwired: 6 in, 3 out]
              }
            }
          }
          frame "ação 2" {
            n155 = call <vilib>:"WPI_RobotDriveTankDrive.vi"("Right axis value"=0.0 ("Left axis value"), "Left axis value"=0.0, "RobotDriveDevRef"=w361) -> ()  [unwired: 6 in, 3 out]
          }
          frame "ação 3" {
            n156 = local read item#7() -> (w368:dbl)
            n157 = Greater?(x=w368, y=18.5) -> (0:w372:bool)
            n158 = call <vilib>:"WPI_RobotDriveTankDrive.vi"("Right axis value"=0.5 ("Left axis value"), "Left axis value"=0.5, "RobotDriveDevRef"=w369) -> ()  [unwired: 6 in, 3 out]
            n159 = case shown="True" w372 {
              tunnel: [T4."ação 3" T4."ação 4"] -> w367
              tunnel: w366 -> [_ w376]
              frame False {
              }
              frame True {
                n160 = call <vilib>:"SPARK Set Sensor Position.vi"("Position"=0.0, "MotorControlDeviceRef"=w376) -> ()  [unwired: 8 in, 2 out]
              }
            }
          }
          frame "ação 4" {
            n161 = local read item#7() -> (w381:dbl)
            n162 = call <vilib>:"WPI_RobotDriveTankDrive.vi"("Right axis value"=-0.5 ("Left axis value"), "Left axis value"=0.5, "RobotDriveDevRef"=w382) -> ()  [unwired: 6 in, 3 out]
            n163 = Less?(x=w381, y=-8.5) -> (x < y?=w384:bool)
            n164 = case shown="True" w384 {
              tunnel: [T4."ação 4" T4."ação 5"] -> w380
              tunnel: w379 -> [_ w389]
              frame False {
              }
              frame True {
                n165 = call <vilib>:"SPARK Set Sensor Position.vi"("Position"=0.0, "MotorControlDeviceRef"=w389) -> ()  [unwired: 8 in, 2 out]
              }
            }
          }
          frame "ação 5" {
            n166 = local read item#7() -> (w394:dbl)
            n167 = call <vilib>:"WPI_RobotDriveTankDrive.vi"("Right axis value"=-0.5 ("Left axis value"), "Left axis value"=-0.5, "RobotDriveDevRef"=w392) -> ("RobotDriveDevRef"=w396:T5)  [unwired: 6 in, 2 out]
            n168 = Less?(x=w394, y=-13.0) -> (x < y?=w395:bool)
            n169 = case shown="True" w395 {
              tunnel: w396 -> [_ w400]
              frame False {
              }
              frame True {
                n170 = call <vilib>:"WPI_RobotDriveTankDrive.vi"("Right axis value"=0.0 ("Left axis value"), "Left axis value"=0.0, "RobotDriveDevRef"=w400) -> ()  [unwired: 6 in, 3 out]
              }
            }
          }
        }
        n171 = Wait (ms)(milliseconds to wait=u32 20) -> ()  [unwired: 1 out]
      }
    }
    frame "meiold" {
      n172 = call <vilib>:"WPI_RobotDriveRefNum Registry Get.vi"("refnum name"="tracao") -> ("error out"=w423:errorcluster, "RobotDriveDevRef"=w422:T5)  [unwired: 9 in]
      n173 = call <vilib>:"WPI_RobotDriveRefNum Registry Get.vi"("refnum name"="rd") -> ("RobotDriveDevRef"=w412:T5)  [unwired: 9 in, 1 out]
      n174 = call <vilib>:"WPI_RobotDriveSafetyConfig.vi"("error in (no error)"=w423, "mode"=WPI_SafetyOutputConfigMenu."Enable", "RobotDriveDevRef"=w422) -> ("RobotDriveDevRef"=w410:T5)  [unwired: 7 in, 1 out]
      n175 = call <vilib>:"WPI_RobotDriveSafetyConfig.vi"("mode"=WPI_SafetyOutputConfigMenu."Enable", "RobotDriveDevRef"=w412) -> ("RobotDriveDevRef"=w411:T5)  [unwired: 8 in, 1 out]
      n176 = Unbundle By Name(w410) -> ("Motors[]"=w421:T6[])
      n177 = Index Array(array=w421) -> (element #1=w414:T6, element #2=w418:T6, element #3=w417:T6, element #4=w416:T6)  [unwired: 4 in]
      n178 = call <vilib>:"SPARK Set Idle Mode.vi"("Idle Mode"=Spark_MAX_Idle_Mode."Brake", "MotorControlDeviceRef in"=w414) -> ()  [unwired: 8 in, 2 out]
      n179 = call <vilib>:"SPARK Set Idle Mode.vi"("Idle Mode"=Spark_MAX_Idle_Mode."Brake", "MotorControlDeviceRef in"=w418) -> ()  [unwired: 8 in, 2 out]
      n180 = call <vilib>:"SPARK Set Idle Mode.vi"("Idle Mode"=Spark_MAX_Idle_Mode."Brake", "MotorControlDeviceRef in"=w417) -> ()  [unwired: 8 in, 2 out]
      n181 = call <vilib>:"SPARK Set Idle Mode.vi"("Idle Mode"=Spark_MAX_Idle_Mode."Brake", "MotorControlDeviceRef in"=w416) -> ()  [unwired: 8 in, 2 out]
      n182 = call <vilib>:"SPARK Set Sensor Position.vi"("Position"=0.0, "MotorControlDeviceRef"=w414) -> ("MotorControlDeviceRef"=w409:T6)  [unwired: 8 in, 1 out]
      n183 = while {
        shift-right: [w432] -> _
        shift-left: T2."ação 1" -> [w434]
        tunnel: w411 -> [w433]
        tunnel: w410 -> [w431]
        tunnel: w409 -> [w429]
        stop <- w427 stop-if-true
        n184 = call <vilib>:"SPARK Get Sensor Position.vi"("MotorControlDevRef in"=w429) -> ("Sensor Position"=→"Sensor Position 2":dbl, "MotorControlDevRef out"=w428:T6)  [unwired: 7 in, 2 out]
        n185 = case shown="\"ação 1\", Default" w434 {
          tunnel: w433 -> [w442 w459 _ _ _ _ _]
          tunnel: [w440 T2."ação 3" w461 w474 w487 w501 T2."ação 8"] -> w432
          tunnel: w431 -> [_ _ w468 w481 w491 w507 w519]
          tunnel: w428 -> [_ _ w462 w475 w494 w502 _]
          tunnel: [FALSE FALSE FALSE FALSE FALSE FALSE w513] -> w427
          frame "ação 1", Default {
            n186 = local read "Numeric 2"() -> (w437:i32)
            n187 = call <vilib>:"WPI_RobotDriveTankDrive.vi"("Right axis value"=1.0, "Left axis value"=0.0, "RobotDriveDevRef"=w442) -> ("RobotDriveDevRef"=w441:T5)  [unwired: 6 in, 2 out]
            n188 = Greater?(x=w437, y=2) -> (0:w436:bool)
            n189 = case shown="True" w436 {
              tunnel: w441 -> [_ w450]
              tunnel: [T2."ação 1" w446] -> w440
              frame False {
              }
              frame True {
                n190 = local read "Numeric 2"() -> (w449:i32)
                n191 = call <vilib>:"WPI_RobotDriveTankDrive.vi"("Right axis value"=1.0 ("Left axis value"), "Left axis value"=1.0 ("Right axis value"), "RobotDriveDevRef"=w450) -> ()  [unwired: 6 in, 3 out]
                n192 = Greater?(x=w449, y=3) -> (0:w447:bool)
                n193 = case shown="False" w447 {
                  tunnel: [T2."ação 1" T2."ação 2"] -> w446
                  frame False {
                  }
                  frame True {
                  }
                }
              }
            }
          }
          frame "ação 2" {
            n194 = call <vilib>:"WPI_RobotDriveTankDrive.vi"("Right axis value"=0.0, "Left axis value"=0.0, "RobotDriveDevRef"=w459) -> ()  [unwired: 6 in, 3 out]
          }
          frame "ação 3" {
            n195 = local read "Sensor Position 2"() -> (w464:dbl)
            n196 = Greater?(x=w464, y=10.0) -> (0:w465:bool)
            n197 = call <vilib>:"WPI_RobotDriveTankDrive.vi"("Right axis value"=0.5 ("Left axis value"), "Left axis value"=0.5, "RobotDriveDevRef"=w468) -> ()  [unwired: 6 in, 3 out]
            n198 = case shown="True" w465 {
              tunnel: w462 -> [_ w472]
              tunnel: [T2."ação 3" T2."ação 4"] -> w461
              frame False {
              }
              frame True {
                n199 = call <vilib>:"SPARK Set Sensor Position.vi"("Position"=0.0, "MotorControlDeviceRef"=w472) -> ()  [unwired: 8 in, 2 out]
              }
            }
          }
          frame "ação 4" {
            n200 = local read "Sensor Position 2"() -> (w478:dbl)
            n201 = call <vilib>:"WPI_RobotDriveTankDrive.vi"("Right axis value"=0.5 ("Left axis value"), "Left axis value"=-0.5, "RobotDriveDevRef"=w481) -> ()  [unwired: 6 in, 3 out]
            n202 = Less?(x=w478, y=-6.0) -> (x < y?=w476:bool)
            n203 = case shown="False" w476 {
              tunnel: w475 -> [_ w485]
              tunnel: [T2."ação 4" T2."ação 5"] -> w474
              frame False {
              }
              frame True {
                n204 = call <vilib>:"SPARK Set Sensor Position.vi"("Position"=0.0, "MotorControlDeviceRef"=w485) -> ()  [unwired: 8 in, 2 out]
              }
            }
          }
          frame "ação 5" {
            n205 = local read "Sensor Position 2"() -> (w490:dbl)
            n206 = call <vilib>:"WPI_RobotDriveTankDrive.vi"("Right axis value"=-0.5 ("Left axis value"), "Left axis value"=-0.5, "RobotDriveDevRef"=w491) -> ()  [unwired: 6 in, 3 out]
            n207 = Less?(x=w490, y=-13.0) -> (x < y?=w488:bool)
            n208 = case shown="True" w488 {
              tunnel: w494 -> [_ w497]
              tunnel: [T2."ação 5" T2."ação 7"] -> w487
              frame False {
              }
              frame True {
                n209 = call <vilib>:"SPARK Set Sensor Position.vi"("Position"=0.0, "MotorControlDeviceRef"=w497) -> ()  [unwired: 8 in, 2 out]
              }
            }
          }
          frame "ação 7" {
            n210 = local read "Sensor Position 2"() -> (w504:dbl)
            n211 = call <vilib>:"WPI_RobotDriveTankDrive.vi"("Right axis value"=0.5 ("Left axis value"), "Left axis value"=-0.5, "RobotDriveDevRef"=w507) -> ()  [unwired: 6 in, 3 out]
            n212 = Less?(x=w504, y=-9.0) -> (x < y?=w503:bool)
            n213 = case shown="True" w503 {
              tunnel: w502 -> [_ w511]
              tunnel: [T2."ação 7" T2."ação 8"] -> w501
              frame False {
              }
              frame True {
                n214 = call <vilib>:"SPARK Set Sensor Position.vi"("Position"=0.0, "MotorControlDeviceRef"=w511) -> ()  [unwired: 8 in, 2 out]
              }
            }
          }
          frame "ação 8" {
            n215 = local read "Sensor Position 2"() -> (w516:dbl)
            n216 = call <vilib>:"WPI_RobotDriveTankDrive.vi"("Right axis value"=-0.5 ("Left axis value"), "Left axis value"=-0.5, "RobotDriveDevRef"=w519) -> ("RobotDriveDevRef"=w514:T5)  [unwired: 6 in, 2 out]
            n217 = Less?(x=w516, y=-45.0) -> (x < y?=w513:bool)
            n218 = case shown="True" w513 {
              tunnel: w514 -> [_ w522]
              frame False {
              }
              frame True {
                n219 = call <vilib>:"WPI_RobotDriveTankDrive.vi"("Right axis value"=0.0 ("Left axis value"), "Left axis value"=0.0, "RobotDriveDevRef"=w522) -> ()  [unwired: 6 in, 3 out]
              }
            }
          }
        }
        n220 = Wait (ms)(milliseconds to wait=u32 20) -> ()  [unwired: 1 out]
      }
      n221 = for {
        N: "Numeric" -> [_]
        i -> [w425]
        n222 = Wait (ms)(milliseconds to wait=u32 1000) -> ()  [unwired: 1 out]
        "Numeric 2" <- w425
      }
    }
    frame "meio ld azul" {
      n223 = call <vilib>:"WPI_RobotDriveRefNum Registry Get.vi"("refnum name"="tracao") -> ("error out"=w542:errorcluster, "RobotDriveDevRef"=w541:T5)  [unwired: 9 in]
      n224 = call <vilib>:"WPI_RobotDriveRefNum Registry Get.vi"("refnum name"="rd") -> ("RobotDriveDevRef"=w531:T5)  [unwired: 9 in, 1 out]
      n225 = call <vilib>:"WPI_RobotDriveSafetyConfig.vi"("error in (no error)"=w542, "mode"=WPI_SafetyOutputConfigMenu."Enable", "RobotDriveDevRef"=w541) -> ("RobotDriveDevRef"=w529:T5)  [unwired: 7 in, 1 out]
      n226 = call <vilib>:"WPI_RobotDriveSafetyConfig.vi"("mode"=WPI_SafetyOutputConfigMenu."Enable", "RobotDriveDevRef"=w531) -> ("RobotDriveDevRef"=w530:T5)  [unwired: 8 in, 1 out]
      n227 = Unbundle By Name(w529) -> ("Motors[]"=w540:T6[])
      n228 = Index Array(array=w540) -> (element #1=w533:T6, element #2=w537:T6, element #3=w536:T6, element #4=w535:T6)  [unwired: 4 in]
      n229 = call <vilib>:"SPARK Set Idle Mode.vi"("Idle Mode"=Spark_MAX_Idle_Mode."Brake", "MotorControlDeviceRef in"=w533) -> ()  [unwired: 8 in, 2 out]
      n230 = call <vilib>:"SPARK Set Idle Mode.vi"("Idle Mode"=Spark_MAX_Idle_Mode."Brake", "MotorControlDeviceRef in"=w537) -> ()  [unwired: 8 in, 2 out]
      n231 = call <vilib>:"SPARK Set Idle Mode.vi"("Idle Mode"=Spark_MAX_Idle_Mode."Brake", "MotorControlDeviceRef in"=w536) -> ()  [unwired: 8 in, 2 out]
      n232 = call <vilib>:"SPARK Set Idle Mode.vi"("Idle Mode"=Spark_MAX_Idle_Mode."Brake", "MotorControlDeviceRef in"=w535) -> ()  [unwired: 8 in, 2 out]
      n233 = call <vilib>:"SPARK Set Sensor Position.vi"("Position"=0.0, "MotorControlDeviceRef"=w533) -> ("MotorControlDeviceRef"=w528:T6)  [unwired: 8 in, 1 out]
      n234 = while {
        shift-right: [w549] -> _
        shift-left: T2."ação 1" -> [w551]
        tunnel: w530 -> [w550]
        tunnel: w529 -> [w548]
        tunnel: w528 -> [w546]
        stop <- w544 stop-if-true
        n235 = call <vilib>:"SPARK Get Sensor Position.vi"("MotorControlDevRef in"=w546) -> ("Sensor Position"=→"Sensor Position 5":dbl, "MotorControlDevRef out"=w545:T6)  [unwired: 7 in, 2 out]
        n236 = case shown="\"ação 1\", Default" w551 {
          tunnel: w550 -> [w559 w571 _ _ _ _ _]
          tunnel: [w554 T2."ação 3" w573 w586 w599 w612 T2."ação 8"] -> w549
          tunnel: w548 -> [_ _ w580 w593 w603 w619 w631]
          tunnel: w545 -> [_ _ w574 w587 w606 w613 _]
          tunnel: [FALSE FALSE FALSE FALSE FALSE FALSE w625] -> w544
          frame "ação 1", Default {
            n237 = Tick Count (ms)() -> (millisecond timer value=w557:u32)
            n238 = call <vilib>:"WPI_RobotDriveTankDrive.vi"("Right axis value"=1.0, "Left axis value"=0.0, "RobotDriveDevRef"=w559) -> ("RobotDriveDevRef"=w558:T5)  [unwired: 6 in, 2 out]
            n239 = Greater?(x=w557, y=u32 1000) -> (0:w555:bool)
            n240 = case shown="True" w555 {
              tunnel: w558 -> [_ w564]
              tunnel: [T2."ação 1" T2."ação 2"] -> w554
              frame False {
              }
              frame True {
                n241 = call <vilib>:"WPI_RobotDriveTankDrive.vi"("Right axis value"=1.0 ("Left axis value"), "Left axis value"=1.0 ("Right axis value"), "RobotDriveDevRef"=w564) -> ()  [unwired: 6 in, 3 out]
              }
            }
          }
          frame "ação 2" {
            n242 = call <vilib>:"WPI_RobotDriveTankDrive.vi"("Right axis value"=0.0, "Left axis value"=0.0, "RobotDriveDevRef"=w571) -> ()  [unwired: 6 in, 3 out]
          }
          frame "ação 3" {
            n243 = local read "Sensor Position 5"() -> (w576:dbl)
            n244 = Greater?(x=w576, y=10.0) -> (0:w577:bool)
            n245 = call <vilib>:"WPI_RobotDriveTankDrive.vi"("Right axis value"=0.5 ("Left axis value"), "Left axis value"=0.5, "RobotDriveDevRef"=w580) -> ()  [unwired: 6 in, 3 out]
            n246 = case shown="True" w577 {
              tunnel: w574 -> [_ w584]
              tunnel: [T2."ação 3" T2."ação 4"] -> w573
              frame False {
              }
              frame True {
                n247 = call <vilib>:"SPARK Set Sensor Position.vi"("Position"=0.0, "MotorControlDeviceRef"=w584) -> ()  [unwired: 8 in, 2 out]
              }
            }
          }
          frame "ação 4" {
            n248 = local read "Sensor Position 5"() -> (w590:dbl)
            n249 = call <vilib>:"WPI_RobotDriveTankDrive.vi"("Right axis value"=0.5 ("Left axis value"), "Left axis value"=-0.5, "RobotDriveDevRef"=w593) -> ()  [unwired: 6 in, 3 out]
            n250 = Greater?(x=w590, y=10.0) -> (0:w588:bool)
            n251 = case shown="True" w588 {
              tunnel: w587 -> [_ w597]
              tunnel: [T2."ação 4" T2."ação 5"] -> w586
              frame False {
              }
              frame True {
                n252 = call <vilib>:"SPARK Set Sensor Position.vi"("Position"=0.0, "MotorControlDeviceRef"=w597) -> ()  [unwired: 8 in, 2 out]
              }
            }
          }
          frame "ação 5" {
            n253 = local read "Sensor Position 5"() -> (w602:dbl)
            n254 = call <vilib>:"WPI_RobotDriveTankDrive.vi"("Right axis value"=-0.5 ("Left axis value"), "Left axis value"=-0.5, "RobotDriveDevRef"=w603) -> ()  [unwired: 6 in, 3 out]
            n255 = Less?(x=w602, y=-13.0) -> (x < y?=w600:bool)
            n256 = case shown="True" w600 {
              tunnel: w606 -> [_ w609]
              tunnel: [T2."ação 5" T2."ação 7"] -> w599
              frame False {
              }
              frame True {
                n257 = call <vilib>:"SPARK Set Sensor Position.vi"("Position"=0.0, "MotorControlDeviceRef"=w609) -> ()  [unwired: 8 in, 2 out]
              }
            }
          }
          frame "ação 7" {
            n258 = local read "Sensor Position 5"() -> (w616:dbl)
            n259 = call <vilib>:"WPI_RobotDriveTankDrive.vi"("Right axis value"=0.5 ("Left axis value"), "Left axis value"=-0.5, "RobotDriveDevRef"=w619) -> ()  [unwired: 6 in, 3 out]
            n260 = Greater?(x=w616, y=10.0) -> (0:w614:bool)
            n261 = case shown="True" w614 {
              tunnel: w613 -> [_ w623]
              tunnel: [T2."ação 7" T2."ação 8"] -> w612
              frame False {
              }
              frame True {
                n262 = call <vilib>:"SPARK Set Sensor Position.vi"("Position"=0.0, "MotorControlDeviceRef"=w623) -> ()  [unwired: 8 in, 2 out]
              }
            }
          }
          frame "ação 8" {
            n263 = local read "Sensor Position 5"() -> (w628:dbl)
            n264 = call <vilib>:"WPI_RobotDriveTankDrive.vi"("Right axis value"=-0.5 ("Left axis value"), "Left axis value"=-0.5, "RobotDriveDevRef"=w631) -> ("RobotDriveDevRef"=w626:T5)  [unwired: 6 in, 2 out]
            n265 = Less?(x=w628, y=-100.0) -> (x < y?=w625:bool)
            n266 = case shown="True" w625 {
              tunnel: w626 -> [_ w634]
              frame False {
              }
              frame True {
                n267 = call <vilib>:"WPI_RobotDriveTankDrive.vi"("Right axis value"=0.0 ("Left axis value"), "Left axis value"=0.0, "RobotDriveDevRef"=w634) -> ()  [unwired: 6 in, 3 out]
              }
            }
          }
        }
        n268 = Wait (ms)(milliseconds to wait=u32 20) -> ()  [unwired: 1 out]
      }
    }
    frame "esquerda" {
      n269 = call <vilib>:"WPI_RobotDriveRefNum Registry Get.vi"("refnum name"="rd") -> ("RobotDriveDevRef"=w644:T5)  [unwired: 9 in, 1 out]
      n270 = call <vilib>:"WPI_RobotDriveRefNum Registry Get.vi"("refnum name"="tracao") -> ("error out"=w654:errorcluster, "RobotDriveDevRef"=w653:T5)  [unwired: 9 in]
      n271 = call <vilib>:"WPI_RobotDriveSafetyConfig.vi"("error in (no error)"=w654, "mode"=WPI_SafetyOutputConfigMenu."Enable", "RobotDriveDevRef"=w653) -> ("RobotDriveDevRef"=w642:T5)  [unwired: 7 in, 1 out]
      n272 = call <vilib>:"WPI_RobotDriveSafetyConfig.vi"("mode"=WPI_SafetyOutputConfigMenu."Enable", "RobotDriveDevRef"=w644) -> ("RobotDriveDevRef"=w643:T5)  [unwired: 8 in, 1 out]
      n273 = Unbundle By Name(w642) -> ("Motors[]"=w652:T6[])
      n274 = Index Array(array=w652) -> (element #1=w646:T6, element #2=w650:T6, element #3=w649:T6, element #4=w648:T6)  [unwired: 4 in]
      n275 = call <vilib>:"SPARK Set Idle Mode.vi"("Idle Mode"=Spark_MAX_Idle_Mode."Brake", "MotorControlDeviceRef in"=w646) -> ()  [unwired: 8 in, 2 out]
      n276 = call <vilib>:"SPARK Set Idle Mode.vi"("Idle Mode"=Spark_MAX_Idle_Mode."Brake", "MotorControlDeviceRef in"=w650) -> ()  [unwired: 8 in, 2 out]
      n277 = call <vilib>:"SPARK Set Idle Mode.vi"("Idle Mode"=Spark_MAX_Idle_Mode."Brake", "MotorControlDeviceRef in"=w649) -> ()  [unwired: 8 in, 2 out]
      n278 = call <vilib>:"SPARK Set Idle Mode.vi"("Idle Mode"=Spark_MAX_Idle_Mode."Brake", "MotorControlDeviceRef in"=w648) -> ()  [unwired: 8 in, 2 out]
      n279 = call <vilib>:"SPARK Set Sensor Position.vi"("Position"=0.0, "MotorControlDeviceRef"=w646) -> ("MotorControlDeviceRef"=w641:T6)  [unwired: 8 in, 1 out]
      n280 = while {
        shift-right: [w656] -> _
        shift-left: T4."ação 1" -> [w657]
        tunnel: w643 -> [w663]
        tunnel: w642 -> [w662]
        tunnel: w641 -> [w660]
        stop <- w658 stop-if-true
        n281 = call <vilib>:"SPARK Get Sensor Position.vi"("MotorControlDevRef in"=w660) -> ("Sensor Position"=→"Sensor Position 3":dbl, "MotorControlDevRef out"=w659:T6)  [unwired: 7 in, 2 out]
        n282 = case shown="\"ação 4\"" w657 {
          tunnel: w663 -> [w669 w683 _ _ _]
          tunnel: w662 -> [_ _ w692 w705 w715]
          tunnel: w659 -> [_ _ w686 w699 _]
          tunnel: [FALSE FALSE FALSE FALSE w710] -> w658
          tunnel: [w670 T4."ação 3" w684 w697 T4."ação 5"] -> w656
          frame "ação 1", Default {
            n283 = Tick Count (ms)() -> (millisecond timer value=w667:u32)
            n284 = call <vilib>:"WPI_RobotDriveTankDrive.vi"("Right axis value"=1.0, "Left axis value"=0.0, "RobotDriveDevRef"=w669) -> ("RobotDriveDevRef"=w668:T5)  [unwired: 6 in, 2 out]
            n285 = Greater?(x=w667, y=u32 3000) -> (0:w665:bool)
            n286 = case shown="True" w665 {
              tunnel: w668 -> [_ w676]
              tunnel: [T4."ação 1" T4."ação 2"] -> w670
              frame False {
              }
              frame True {
                n287 = call <vilib>:"WPI_RobotDriveTankDrive.vi"("Right axis value"=1.0 ("Left axis value"), "Left axis value"=1.0 ("Right axis value"), "RobotDriveDevRef"=w676) -> ()  [unwired: 6 in, 3 out]
              }
            }
          }
          frame "ação 2" {
            n288 = call <vilib>:"WPI_RobotDriveTankDrive.vi"("Right axis value"=0.0, "Left axis value"=0.0, "RobotDriveDevRef"=w683) -> ()  [unwired: 6 in, 3 out]
          }
          frame "ação 3" {
            n289 = local read "Sensor Position 3"() -> (w688:dbl)
            n290 = Greater?(x=w688, y=57.0) -> (0:w689:bool)
            n291 = call <vilib>:"WPI_RobotDriveTankDrive.vi"("Right axis value"=0.5 ("Left axis value"), "Left axis value"=0.5, "RobotDriveDevRef"=w692) -> ()  [unwired: 6 in, 3 out]
            n292 = case shown="True" w689 {
              tunnel: w686 -> [_ w696]
              tunnel: [T4."ação 3" T4."ação 4"] -> w684
              frame False {
              }
              frame True {
                n293 = call <vilib>:"SPARK Set Sensor Position.vi"("Position"=0.0, "MotorControlDeviceRef"=w696) -> ()  [unwired: 8 in, 2 out]
              }
            }
          }
          frame "ação 4" {
            n294 = local read "Sensor Position 3"() -> (w702:dbl)
            n295 = call <vilib>:"WPI_RobotDriveTankDrive.vi"("Right axis value"=0.5 ("Left axis value"), "Left axis value"=-0.5, "RobotDriveDevRef"=w705) -> ()  [unwired: 6 in, 3 out]
            n296 = Less?(x=w702, y=-8.0) -> (x < y?=w700:bool)
            n297 = case shown="True" w700 {
              tunnel: w699 -> [_ w709]
              tunnel: [T4."ação 4" T4."ação 5"] -> w697
              frame False {
              }
              frame True {
                n298 = call <vilib>:"SPARK Set Sensor Position.vi"("Position"=0.0, "MotorControlDeviceRef"=w709) -> ()  [unwired: 8 in, 2 out]
              }
            }
          }
          frame "ação 5" {
            n299 = local read "Sensor Position 3"() -> (w714:dbl)
            n300 = call <vilib>:"WPI_RobotDriveTankDrive.vi"("Right axis value"=-0.5 ("Left axis value"), "Left axis value"=-0.5, "RobotDriveDevRef"=w715) -> ("RobotDriveDevRef"=w712:T5)  [unwired: 6 in, 2 out]
            n301 = Less?(x=w714, y=-60.0) -> (x < y?=w710:bool)
            n302 = case shown="True" w710 {
              tunnel: w712 -> [_ w718]
              frame False {
              }
              frame True {
                n303 = call <vilib>:"WPI_RobotDriveTankDrive.vi"("Right axis value"=0.0 ("Left axis value"), "Left axis value"=0.0, "RobotDriveDevRef"=w718) -> ()  [unwired: 6 in, 3 out]
              }
            }
          }
        }
        n304 = Wait (ms)(milliseconds to wait=u32 20) -> ()  [unwired: 1 out]
      }
    }
    frame "esquerdaazul" {
      n305 = call <vilib>:"WPI_RobotDriveRefNum Registry Get.vi"("refnum name"="rd") -> ("RobotDriveDevRef"=w730:T5)  [unwired: 9 in, 1 out]
      n306 = call <vilib>:"WPI_RobotDriveRefNum Registry Get.vi"("refnum name"="tracao") -> ("error out"=w740:errorcluster, "RobotDriveDevRef"=w739:T5)  [unwired: 9 in]
      n307 = call <vilib>:"WPI_RobotDriveSafetyConfig.vi"("error in (no error)"=w740, "mode"=WPI_SafetyOutputConfigMenu."Enable", "RobotDriveDevRef"=w739) -> ("RobotDriveDevRef"=w728:T5)  [unwired: 7 in, 1 out]
      n308 = call <vilib>:"WPI_RobotDriveSafetyConfig.vi"("mode"=WPI_SafetyOutputConfigMenu."Enable", "RobotDriveDevRef"=w730) -> ("RobotDriveDevRef"=w729:T5)  [unwired: 8 in, 1 out]
      n309 = Unbundle By Name(w728) -> ("Motors[]"=w738:T6[])
      n310 = Index Array(array=w738) -> (element #1=w732:T6, element #2=w736:T6, element #3=w735:T6, element #4=w734:T6)  [unwired: 4 in]
      n311 = call <vilib>:"SPARK Set Idle Mode.vi"("Idle Mode"=Spark_MAX_Idle_Mode."Brake", "MotorControlDeviceRef in"=w732) -> ()  [unwired: 8 in, 2 out]
      n312 = call <vilib>:"SPARK Set Idle Mode.vi"("Idle Mode"=Spark_MAX_Idle_Mode."Brake", "MotorControlDeviceRef in"=w736) -> ()  [unwired: 8 in, 2 out]
      n313 = call <vilib>:"SPARK Set Idle Mode.vi"("Idle Mode"=Spark_MAX_Idle_Mode."Brake", "MotorControlDeviceRef in"=w735) -> ()  [unwired: 8 in, 2 out]
      n314 = call <vilib>:"SPARK Set Idle Mode.vi"("Idle Mode"=Spark_MAX_Idle_Mode."Brake", "MotorControlDeviceRef in"=w734) -> ()  [unwired: 8 in, 2 out]
      n315 = call <vilib>:"SPARK Set Sensor Position.vi"("Position"=0.0, "MotorControlDeviceRef"=w732) -> ("MotorControlDeviceRef"=w727:T6)  [unwired: 8 in, 1 out]
      n316 = while {
        shift-right: [w742] -> _
        shift-left: T4."ação 1" -> [w743]
        tunnel: w729 -> [w749]
        tunnel: w728 -> [w748]
        tunnel: w727 -> [w746]
        stop <- w744 stop-if-true
        n317 = call <vilib>:"SPARK Get Sensor Position.vi"("MotorControlDevRef in"=w746) -> ("Sensor Position"=→"Sensor Position 4":dbl, "MotorControlDevRef out"=w745:T6)  [unwired: 7 in, 2 out]
        n318 = case shown="\"ação 4\"" w743 {
          tunnel: w749 -> [w757 w769 _ _ _]
          tunnel: w748 -> [_ _ w778 w791 w801]
          tunnel: w745 -> [_ _ w772 w785 _]
          tunnel: [FALSE FALSE FALSE FALSE w796] -> w744
          tunnel: [w751 T4."ação 3" w770 w783 T4."ação 5"] -> w742
          frame "ação 1", Default {
            n319 = Tick Count (ms)() -> (millisecond timer value=w755:u32)
            n320 = call <vilib>:"WPI_RobotDriveTankDrive.vi"("Right axis value"=1.0, "Left axis value"=0.0, "RobotDriveDevRef"=w757) -> ("RobotDriveDevRef"=w756:T5)  [unwired: 6 in, 2 out]
            n321 = Greater?(x=w755, y=u32 1000) -> (0:w753:bool)
            n322 = case shown="True" w753 {
              tunnel: w756 -> [_ w762]
              tunnel: [T4."ação 1" T4."ação 2"] -> w751
              frame False {
              }
              frame True {
                n323 = call <vilib>:"WPI_RobotDriveTankDrive.vi"("Right axis value"=1.0 ("Left axis value"), "Left axis value"=1.0 ("Right axis value"), "RobotDriveDevRef"=w762) -> ()  [unwired: 6 in, 3 out]
              }
            }
          }
          frame "ação 2" {
            n324 = call <vilib>:"WPI_RobotDriveTankDrive.vi"("Right axis value"=0.0, "Left axis value"=0.0, "RobotDriveDevRef"=w769) -> ()  [unwired: 6 in, 3 out]
          }
          frame "ação 3" {
            n325 = local read "Sensor Position 4"() -> (w774:dbl)
            n326 = Greater?(x=w774, y=57.0) -> (0:w775:bool)
            n327 = call <vilib>:"WPI_RobotDriveTankDrive.vi"("Right axis value"=0.5 ("Left axis value"), "Left axis value"=0.5, "RobotDriveDevRef"=w778) -> ()  [unwired: 6 in, 3 out]
            n328 = case shown="False" w775 {
              tunnel: w772 -> [_ w782]
              tunnel: [T4."ação 3" T4."ação 4"] -> w770
              frame False {
              }
              frame True {
                n329 = call <vilib>:"SPARK Set Sensor Position.vi"("Position"=0.0, "MotorControlDeviceRef"=w782) -> ()  [unwired: 8 in, 2 out]
              }
            }
          }
          frame "ação 4" {
            n330 = local read "Sensor Position 4"() -> (w788:dbl)
            n331 = call <vilib>:"WPI_RobotDriveTankDrive.vi"("Right axis value"=0.5 ("Left axis value"), "Left axis value"=-0.5, "RobotDriveDevRef"=w791) -> ()  [unwired: 6 in, 3 out]
            n332 = Less?(x=w788, y=-10.0) -> (x < y?=w786:bool)
            n333 = case shown="False" w786 {
              tunnel: w785 -> [_ w795]
              tunnel: [T4."ação 4" T4."ação 5"] -> w783
              frame False {
              }
              frame True {
                n334 = call <vilib>:"SPARK Set Sensor Position.vi"("Position"=0.0, "MotorControlDeviceRef"=w795) -> ()  [unwired: 8 in, 2 out]
              }
            }
          }
          frame "ação 5" {
            n335 = local read "Sensor Position 4"() -> (w800:dbl)
            n336 = call <vilib>:"WPI_RobotDriveTankDrive.vi"("Right axis value"=-0.5 ("Left axis value"), "Left axis value"=-0.5, "RobotDriveDevRef"=w801) -> ("RobotDriveDevRef"=w798:T5)  [unwired: 6 in, 2 out]
            n337 = Less?(x=w800, y=-60.0) -> (x < y?=w796:bool)
            n338 = case shown="False" w796 {
              tunnel: w798 -> [_ w804]
              frame False {
              }
              frame True {
                n339 = call <vilib>:"WPI_RobotDriveTankDrive.vi"("Right axis value"=0.0 ("Left axis value"), "Left axis value"=0.0, "RobotDriveDevRef"=w804) -> ()  [unwired: 6 in, 3 out]
              }
            }
          }
        }
        n340 = Wait (ms)(milliseconds to wait=u32 20) -> ()  [unwired: 1 out]
      }
    }
    frame "teste shooter" {
      n341 = call <vilib>:"WPI_RobotDriveRefNum Registry Get.vi"("refnum name"="rd") -> ("RobotDriveDevRef"=w812:T5)  [unwired: 9 in, 1 out]
      n342 = call <vilib>:"WPI_RobotDriveTankDrive.vi"("Right axis value"=1.0 ("Left axis value"), "Left axis value"=1.0, "RobotDriveDevRef"=w812) -> ("RobotDriveDevRef"=w807:T5)  [unwired: 6 in, 2 out]
      n343 = Unbundle By Name(w807) -> ("Motors[]"=w808:T6[])
      n344 = while {
        tunnel: w808 -> [w820]
        stop <- w817 stop-if-true
        n345 = Index Array(array=w820) -> (element #1=w825:T6, element #2=w824:T6)  [unwired: 2 in]
        n346 = Wait (ms)(milliseconds to wait=u32 20) -> ()  [unwired: 1 out]
        n347 = call <vilib>:"SPARK Get Sensor Position.vi"("MotorControlDevRef in"=w824) -> ("Sensor Position"=w823:dbl, "MotorControlDevRef out"=w815:T6)  [unwired: 7 in, 2 out]
        "Sensor Position 7" <- w823
        n348 = call <vilib>:"SPARK Get Sensor Position.vi"("MotorControlDevRef in"=w825) -> ("Sensor Position"=w813:dbl, "MotorControlDevRef out"=w814:T6)  [unwired: 7 in, 2 out]
        "Sensor Position 8" <- w813
        n349 = Greater?(x=w823, y=50.0) -> (0:w818:bool)
        n350 = Greater?(x=w813, y=50.0) -> (0:w819:bool)
        n351 = And(x=w819, y=w818) -> (x .and. y?=w817:bool)
        n352 = case shown="True" w819 {
          tunnel: w814 -> [_ w833]
          frame False {
          }
          frame True {
            n353 = call <vilib>:"WPI_MotorControlSetOutput.vi"("Output"=0.0, "MotorControlDevRef"=w833) -> ("MotorControlDevRef"=w831:T6)  [unwired: 7 in, 2 out]
            n354 = call <vilib>:"SPARK Set Sensor Position.vi"("Position"=0.0, "MotorControlDeviceRef"=w831) -> ()  [unwired: 8 in, 2 out]
          }
        }
        n355 = case shown="True" w818 {
          tunnel: w815 -> [_ w829]
          frame False {
          }
          frame True {
            n356 = call <vilib>:"WPI_MotorControlSetOutput.vi"("Output"=0.0, "MotorControlDevRef"=w829) -> ("MotorControlDevRef"=w827:T6)  [unwired: 7 in, 2 out]
            n357 = call <vilib>:"SPARK Set Sensor Position.vi"("Position"=0.0, "MotorControlDeviceRef"=w827) -> ()  [unwired: 8 in, 2 out]
          }
        }
      }
    }
  }
